vi "PH_Timing.set i attribute.vi"(0 "i ref in":refnum<vi>, 2 "i attribute":T1={"Sequencer"={"linked?"=FALSE, "Proc State"="no info", "Ref State"=refnum}, "Gate Generator"={"GD"={"Device Status"=0, "linked?"=FALSE}, "Settings"={"Instance"="N/A", "Channel Gate"=1, "Channel T2"=1, "Width Gate"=1.0, "Width T2"=1.0, "Delay Gate"=0.0, "Delay T2"=0.0, "Gate activ"=FALSE, "T2 activ"=FALSE, "System Mode"=enum."Normal"}, "GUI Ref"=refnum}, "Interlock Bypass"={"Instancename"="N/A", "Switch linked?"=FALSE, "Device Status"=0, "Ref Status"=refnum}, "Roughtuner"={"Settings"={"Instance"="N/A", "Phase PHELIX / UNILAC"={"Channel"=0, "relative to"=0, "Delay [ms]"=0.0}, "Pulse Length"={"Channel"=0, "relative to"=0, "Delay [ms]"=0.0}, "Trigger"={"externally?"=FALSE, "Rate [Hz]"=0.0}}, "GUI Ref"=refnum, "GD"={"Device Status"=0, "linked?"=FALSE}}, "0,5Hz Gater"={"Settings"={"Instance"="N/A", "Channel ns FE Delay"=1, "Channel 0.5Hz"=1, "Width ns FE Delay"=1.0, "Width 0.5Hz"=1.0, "Delay ns FE Delay"=0.0, "Delay 0.5Hz"=0.0, "ns FE Delay active"=FALSE, "0.5Hz activ"=FALSE, "ns FE Delay inverted"=FALSE, "0.5Hz inverted"=FALSE}, "GUI Ref"=refnum, "GD"={"Device Status"=0, "linked?"=FALSE}}, "Slow Trigger"={"Settings"={"Delay"=0.0, "externally triggered?"=FALSE}, "GUI Ref"=refnum, "Service ID Delay"=-1, "Service ID Ext Trig"=-1, "Wanted Settings"={"Delay"=0.0, "externally triggered?"=FALSE}}, "Timing Mode"={"Mode"={"T2"=0, "Modeselector"=enum."0.5 Hz"}, "GUI Ref"=refnum, "Service ID T2"=-1, "Service ID Mode"=-1, "Wanted Mode"={"T2"=0, "Modeselector"=enum."10 Hz"}}, "ns Generator"={"Settings"={"Instance"="N/A", "Phase fs / ns FE"={"Channel"=0, "Settings"={"Delay [s]"=0.0, "relative to"=0}}}, "ns Generator Settings"=refnum, "GD"={"Device Status"=0, "linked?"=FALSE}}, "Phase FEs"={"Settings"={"Phase"=0.0}, "GUI Ref"=refnum, "Service ID Phase"=-1, "Wanted Settings"={"Phase"=0.0}}, "GD GUI Refs"=[], "Heads"=[], "GUI Ref Delete"=refnum} {"Heads"."GD"."Device Status" items=["no info", "off/false/out", "on/true/in", "Failure", "Alarm", "Status 1", "Status 2", "Status 3"]; "Heads"."Data"."CH" items=["System (To)", "Channel A", "Channel B", "Channel C", "Channel D", "Channel E", "Channel F", "Channel G", "Channel H"]; "Heads"."Data"."Delay" format="%#_7f"; "Phase FEs"."Wanted Settings"."Phase" format="%#_12p"; "Phase FEs"."Settings"."Phase" format="%#_12p"; "ns Generator"."GD"."Device Status" items=["no info", "off/false/out", "on/true/in", "Failure", "Alarm", "Status 1", "Status 2", "Status 3"]; "ns Generator"."Settings"."Phase fs / ns FE"."Settings"."relative to" items=["T0", "T1", "A", "B", "C", "D", "E", "F", "G", "H"]; "ns Generator"."Settings"."Phase fs / ns FE"."Settings"."Delay [s]" format="%#_12p"; "ns Generator"."Settings"."Phase fs / ns FE"."Channel" items=["T0", "T1", "A", "B", "C", "D", "E", "F", "G", "H"]; "Timing Mode"."Wanted Mode"."T2" min=0 max=6000 step=2; "Timing Mode"."Mode"."T2" min=0 max=6000 step=2; "0,5Hz Gater"."GD"."Device Status" items=["no info", "off/false/out", "on/true/in", "Failure", "Alarm", "Status 1", "Status 2", "Status 3"]; "0,5Hz Gater"."Settings"."Channel ns FE Delay" items=["System (To)", "Channel A", "Channel B", "Channel C", "Channel D", "Channel E", "Channel F", "Channel G", "Channel H"]; "0,5Hz Gater"."Settings"."Channel 0.5Hz" items=["System (To)", "Channel A", "Channel B", "Channel C", "Channel D", "Channel E", "Channel F", "Channel G", "Channel H"]; "Roughtuner"."GD"."Device Status" items=["no info", "off/false/out", "on/true/in", "Failure", "Alarm", "Status 1", "Status 2", "Status 3"]; "Roughtuner"."Settings"."Pulse Length"."Delay [ms]" format="%#_8g"; "Roughtuner"."Settings"."Pulse Length"."relative to" items=["T0", "A", "B", "AB", "C", "D", "CD"]; "Roughtuner"."Settings"."Pulse Length"."Channel" items=["T0", "A", "B", "AB", "C", "D", "CD"]; "Roughtuner"."Settings"."Phase PHELIX / UNILAC"."Delay [ms]" format="%#_8g"; "Roughtuner"."Settings"."Phase PHELIX / UNILAC"."relative to" items=["T0", "A", "B", "AB", "C", "D", "CD"]; "Roughtuner"."Settings"."Phase PHELIX / UNILAC"."Channel" items=["T0", "A", "B", "AB", "C", "D", "CD"]; "Interlock Bypass"."Device Status" items=["no info", "off/false/out", "on/true/in", "Failure", "Alarm", "Status 1", "Status 2", "Status 3"]; "Gate Generator"."Settings"."Channel Gate" items=["System (To)", "Channel A", "Channel B", "Channel C", "Channel D", "Channel E", "Channel F", "Channel G", "Channel H"]; "Gate Generator"."Settings"."Channel T2" items=["System (To)", "Channel A", "Channel B", "Channel C", "Channel D", "Channel E", "Channel F", "Channel G", "Channel H"]; "Gate Generator"."GD"."Device Status" items=["no info", "off/false/out", "on/true/in", "Failure", "Alarm", "Status 1", "Status 2", "Status 3"]}, 5 "error in (no error)":errorcluster) -> (14 "i ref out":refnum<vi>, 19 "error out":errorcluster)   [LabVIEW 2014, in "PH_Timing.lvlib"]
doc: "Sets the i attribute data of an object.\n\nLicense Agreement for this software:\n\nCopyright (C)\nGesellschaft für Schwerionenforschung, GSI\nPlanckstr. 1\n64291 Darmstadt\nGermany\n\nContact: D.Beck@gsi.de \n\nThis program is free software; you can redistribute it and/or modify it under the terms of the GNU General Public License as published by the Free Software Foundation; either version 2 of the license, or (at your option) any later version.\n\nThis program is distributed in the hope that it will be useful, but WITHOUT ANY WARRANTY; without even the implied warranty of MERCHANTABILITY or FITNESS FOR A PARTICULAR PURPOSE. See the GNU General License for more details (http://www.gnu.org).\n\nGesellschaft für Schwerionenforschung, GSI\nPlanckstr. 1, 64291 Darmstadt, Germany\nFor all questions and ideas contact: M.Richter@gsi.de, H.Brand@gsi.de or D.Beck@gsi.de.\nLast update: 17-JUN-2004"
uses:
  PH_Timing.lvlib
  PH_Timing.i attribute.ctl
  PH_StatusHandler/PH_StatusHandler.Status.ctl
  PH_Timing.GateGen.ctl
  PH_Timing.Roughtuner.ctl
  PH_Timing.0.5HzGater.ctl
  PH_Timing.Slow Trigger Settings.ctl
  PH_Timing.Timing Mode.ctl
  PH_Timing.ns Generator.ctl
  instr.lib/Stanford Research DG645/Driver/Channel.ctl
  PH_SRDG645/PH_SRDG645.Channel Settings.ctl
  PH_Timing.Phase FEs.ctl
  PH_Timing.PU Data.ctl
  PH_Timing.PU Info.ctl
  PH_PP_Common/PH_PP_Common.PUs.ctl
  PH_StatusHandler/PH_StatusHandler.lvlib
  instr.lib/Stanford Research DG645/Stanford Research DG645 - Driver.lvlib
  PH_SRDG645/PH_SRDG645.lvlib
  PH_PP_Common/PH_PP_Common.lvlib
panel:
  # "s"
  # "s"
  # "AND ns FE Delay"
  # "AND 0.5 Hz"
  # "Gate"
  # "T2"
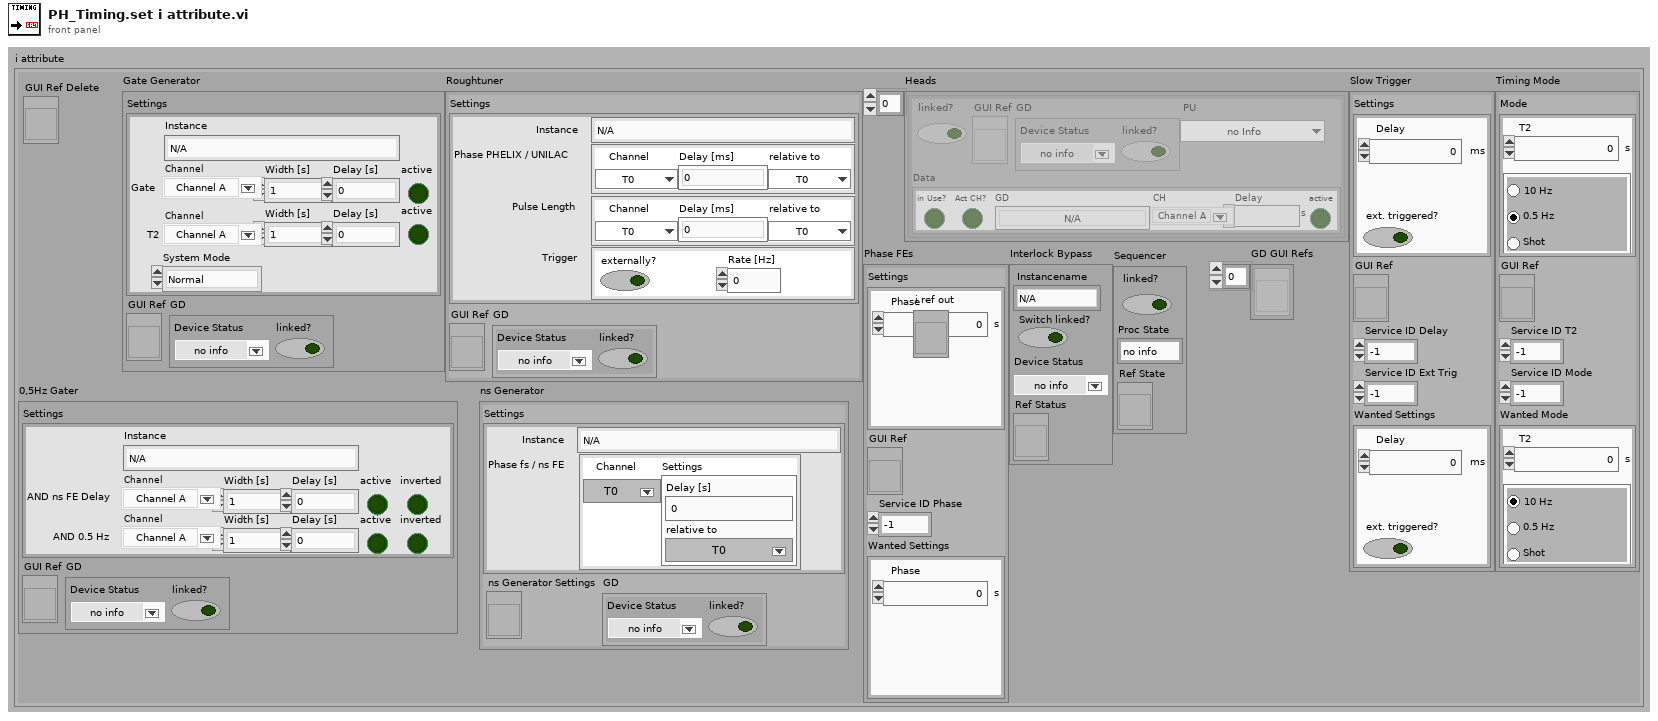
[diagram p1: front panel]
types:
  T1 = typedef "PH_Timing.lvlib/PH_Timing.i attribute.ctl" = cluster{"Sequencer":cluster{"linked?":bool, "Proc State":string, "Ref State":refnum<vi>}, "Gate Generator":cluster{"GD":cluster{"Device Status":T2, "linked?":bool}, "Settings":T3, "GUI Ref":refnum<vi>}, "Interlock Bypass":cluster{"Instancename":string, "Switch linked?":bool, "Device Status":T2, "Ref Status":refnum<vi>}, "Roughtuner":cluster{"Settings":T4, "GUI Ref":refnum<vi>, "GD":cluster{"Device Status":T2, "linked?":bool}}, "0,5Hz Gater":cluster{"Settings":T5, "GUI Ref":refnum<vi>, "GD":cluster{"Device Status":T2, "linked?":bool}}, "Slow Trigger":cluster{"Settings":T6, "GUI Ref":refnum<vi>, "Service ID Delay":i32, "Service ID Ext Trig":i32, "Wanted Settings":T6}, "Timing Mode":cluster{"Mode":T7, "GUI Ref":refnum<vi>, "Service ID T2":i32, "Service ID Mode":i32, "Wanted Mode":T7}, "ns Generator":cluster{"Settings":T8, "ns Generator Settings":refnum<vi>, "GD":cluster{"Device Status":T2, "linked?":bool}}, "Phase FEs":cluster{"Settings":T11, "GUI Ref":refnum<vi>, "Service ID Phase":i32, "Wanted Settings":T11}, "GD GUI Refs":refnum<vi>[], "Heads":T12[], "GUI Ref Delete":refnum<vi>}
  T2 = typedef "PH_StatusHandler.lvlib/PH_StatusHandler.Status.ctl" = i16
  T3 = typedef "PH_Timing.lvlib/PH_Timing.GateGen.ctl" = cluster{"Instance":string, "Channel Gate":i32, "Channel T2":i32, "Width Gate":dbl, "Width T2":dbl, "Delay Gate":dbl, "Delay T2":dbl, "Gate activ":bool, "T2 activ":bool, "System Mode":enum16{"Normal", "Single", "Burst", "Duty Cycle"}}
  T4 = typedef "PH_Timing.lvlib/PH_Timing.Roughtuner.ctl" = cluster{"Instance":string, "Phase PHELIX / UNILAC":cluster{"Channel":u16, "relative to":u16, "Delay [ms]":dbl}, "Pulse Length":cluster{"Channel":u16, "relative to":u16, "Delay [ms]":dbl}, "Trigger":cluster{"externally?":bool, "Rate [Hz]":dbl}}
  T5 = typedef "PH_Timing.lvlib/PH_Timing.0.5HzGater.ctl" = cluster{"Instance":string, "Channel ns FE Delay":i32, "Channel 0.5Hz":i32, "Width ns FE Delay":dbl, "Width 0.5Hz":dbl, "Delay ns FE Delay":dbl, "Delay 0.5Hz":dbl, "ns FE Delay active":bool, "0.5Hz activ":bool, "ns FE Delay inverted":bool, "0.5Hz inverted":bool}
  T6 = typedef "PH_Timing.lvlib/PH_Timing.Slow Trigger Settings.ctl" = cluster{"Delay":dbl, "externally triggered?":bool}
  T7 = typedef "PH_Timing.lvlib/PH_Timing.Timing Mode.ctl" = cluster{"T2":i16, "Modeselector":enum32{"10 Hz", "0.5 Hz", "Shot"}}
  T8 = typedef "PH_Timing.lvlib/PH_Timing.ns Generator.ctl" = cluster{"Instance":string, "Phase fs / ns FE":cluster{"Channel":T9, "Settings":T10}}
  T9 = typedef "Stanford Research DG645 - Driver.lvlib/Channel.ctl" = i32
  T10 = typedef "PH_SRDG645.lvlib/PH_SRDG645.Channel Settings.ctl" = cluster{"Delay [s]":dbl, "relative to":i32}
  T11 = typedef "PH_Timing.lvlib/PH_Timing.Phase FEs.ctl" = cluster{"Phase":dbl}
  T12 = typedef "PH_Timing.lvlib/PH_Timing.PU Data.ctl" = cluster{"linked?":bool, "Data":T13, "GD":cluster{"Device Status":T2, "linked?":bool}, "GUI Ref":refnum<vi>, "PU":T14}
  T13 = typedef "PH_Timing.lvlib/PH_Timing.PU Info.ctl" = cluster{"Act CH?":bool, "GD":string, "CH":i32, "Delay":dbl, "active":bool, "in Use?":bool}
  T14 = typedef "PH_PP_Common.lvlib/PH_PP_Common.PUs.ctl" = enum16{"no Info", "PA-19mm-1", "PA-19mm-2", "PA-45mm-PILC", "PA-45mm-MAIN", "MA-PU-1", "MA-PU-2", "MA-PU-3", "MA-PU-4", "MA-PU-5", "MA-PU-6", "MA-FR", "MA-PILC", "PA-45mm-DP"}
  T15 = enum16{"SetAttribute", "GetAttribute", "CreateAttribute", "DestroyAttribute", "DestroyAllAtributes"}
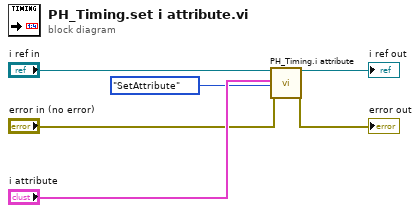
[diagram p0: block diagram]
diagram:
  n1 = call "PH_Timing.i attribute.vi"("VI Refnum"="i ref in", "CLASS.i attribute"="i attribute", "Action"=T15."SetAttribute", "error in (no error)"="error in (no error)") -> ("VI Refnum out"=→"i ref out":refnum<vi>, "error out"=→"error out":errorcluster)  [unwired: 13 in, 1 out]
